vi "LED_control.vi"() -> ()   [LabVIEW 2018]
uses:
  <instrlib>/niDMM/nidmm.llb/niDMM Function.ctl
  <instrlib>/niDMM/nidmm.llb/niDMM Resolution in Digits.ctl
  <instrlib>/niDCPower/nidcpower.llb/niDCPower Measurement Type.ctl
  <vilib>/Instr/_visa.llb/VISA Configure Serial Port (Instr).vi
  <instrlib>/niDMM/nidmm.llb/niDMM Configure Measurement Digits.vi
panel:
  in  "Command":string="led_on"
  in  "Записать":bool
  in  "Tab Control":enum32{"Рабочая область", "Служебная область"}(tab)
  out "Тип индикатора":string
  in  "Питание":bool
  in  "Стоп":bool
  in  "Resource Name":refnum<k15>="PXI1Slot2" caption="Источник питания"
  in  "Мультиметр":refnum<k15>="PXI1Slot5" caption="NI DMM 1"
  in  "V_MB, V":dbl=6.0 caption="voltage level" format="%_6p"
  in  "curlim_V_MB, A":dbl=0.3 caption="current limit" format="%_6p"
  in  "curlim_V_RESERVE, A":dbl=0.1 caption="current limit" format="%_6p"
  out "currentmes_V_MB, A":dbl caption="measurement" format="%_6g"
  out "currentmes_V_RESERVE, A":dbl caption="measurement" format="%_6g"
  in  "V_RESERVE, V":dbl caption="voltage level" format="%_6p"
  out "chart_2":dbl(graph)=8.556104343922883e-07
  out "chart_0":dbl(graph)=5.42616690347781e-05 caption="Waveform Chart 5"
  in  "curlim_V_LED, A":dbl=0.03 caption="current limit" format="%_6p"
  in  "V_LED, V":dbl=2.000000000000001 caption="voltage level" format="%_6p"
  out "chart_1":dbl(graph)=2.456762028615791e-06 caption="Waveform Chart 5"
  out "currentmes_V_LED, A":dbl caption="measurement" format="%_6g"
  in  "NI DMM 1 Current Range 3":string(combo)="0,1" caption="Range"
  out "Real Current, А":dbl=1.3612861948786303e-08 format="%.5f"
  in  "NI DMM 1 units 3":string(combo)="1000" caption="Units"
  out "NI DMM 1 Current Char 3":dbl(graph)=0.013612861948786303
  out "NI DMM 1 Current 3":dbl caption="Current" format="%_6g"
  in  "Arduino":refnum<visa-resource-name>="COM14"
  in  "Сегменты":bool[](array[boolean])=[FALSE, FALSE, FALSE, FALSE, FALSE, FALSE, FALSE, FALSE, FALSE, FALSE]
  out "Разряд":dbl
  out "+/-":bool
  # "all_off - 0\nall_on - 1"
  # "j"
  # "c"
  # "d"
  # "e"
  # "g"
  # "h"
  # "a"
  # "b"
  # "f"
  # "k"
  # "L"
  # "m"
  # "n"
  # "p"
  # "dp"
  # "необходимо выдерживать 1 с между нажатиями кнопок"
  # "регулировать ток в зависимости от температуры.\nс ростом температуры растет ток.\nпид-регулятор??"
  # "\"опрашивать кнопки не чаще, чем раз в секунду. сейчас кликать можно чаще, они загорятся, но ничего не произойдет\""
  # "автоматизировать подбор напряжения по известному максимальному напряжению и току. ОС по току сегмента"
  # "регклировка суммарного тока через инлдикатор"
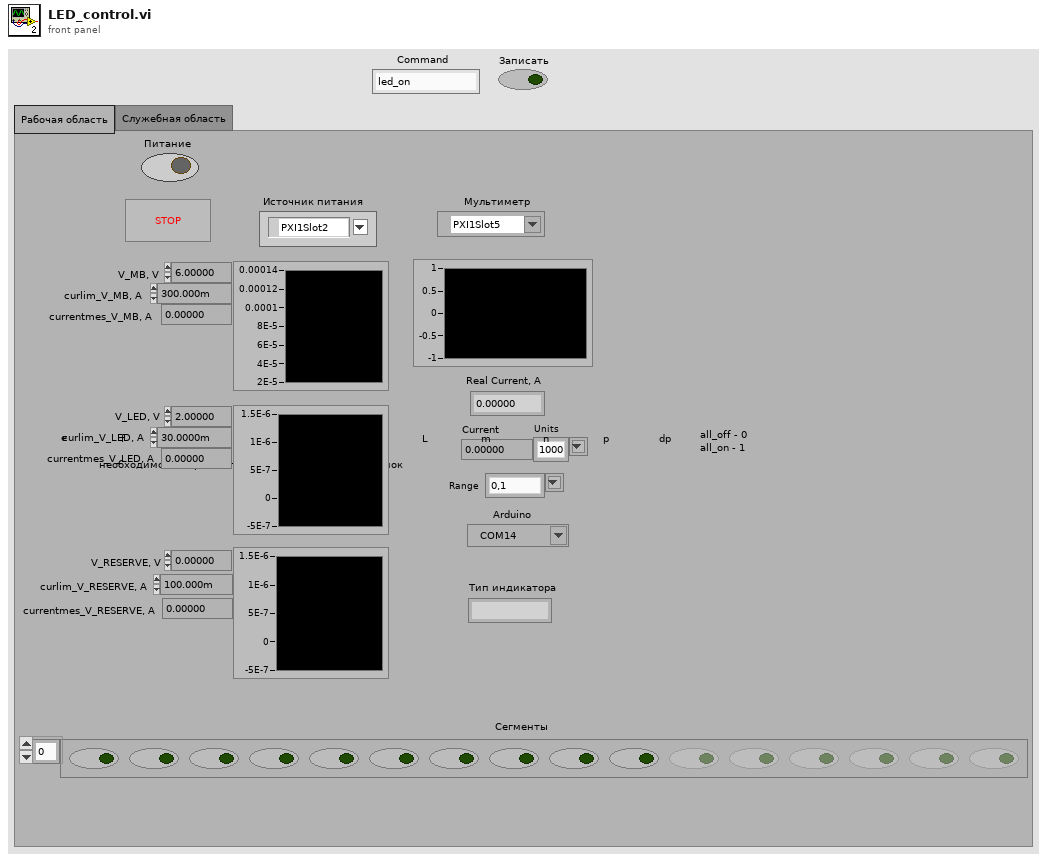
[diagram p1: front panel]
types:
  T1 = typedef "niDMM Function.ctl" = enum16{"DC Volts", "AC Volts", "DC Current", "AC Current", "2-wire Resistance", "4-wire Resistance", "Diode", "Frequency", "Period", "AC Volts DC Coupled", "Capacitance", "Inductance", "Temperature"}
  T2 = typedef "niDMM Resolution in Digits.ctl" = dbl
  T3 = typedef "niDCPower Measurement Type.ctl" = i32
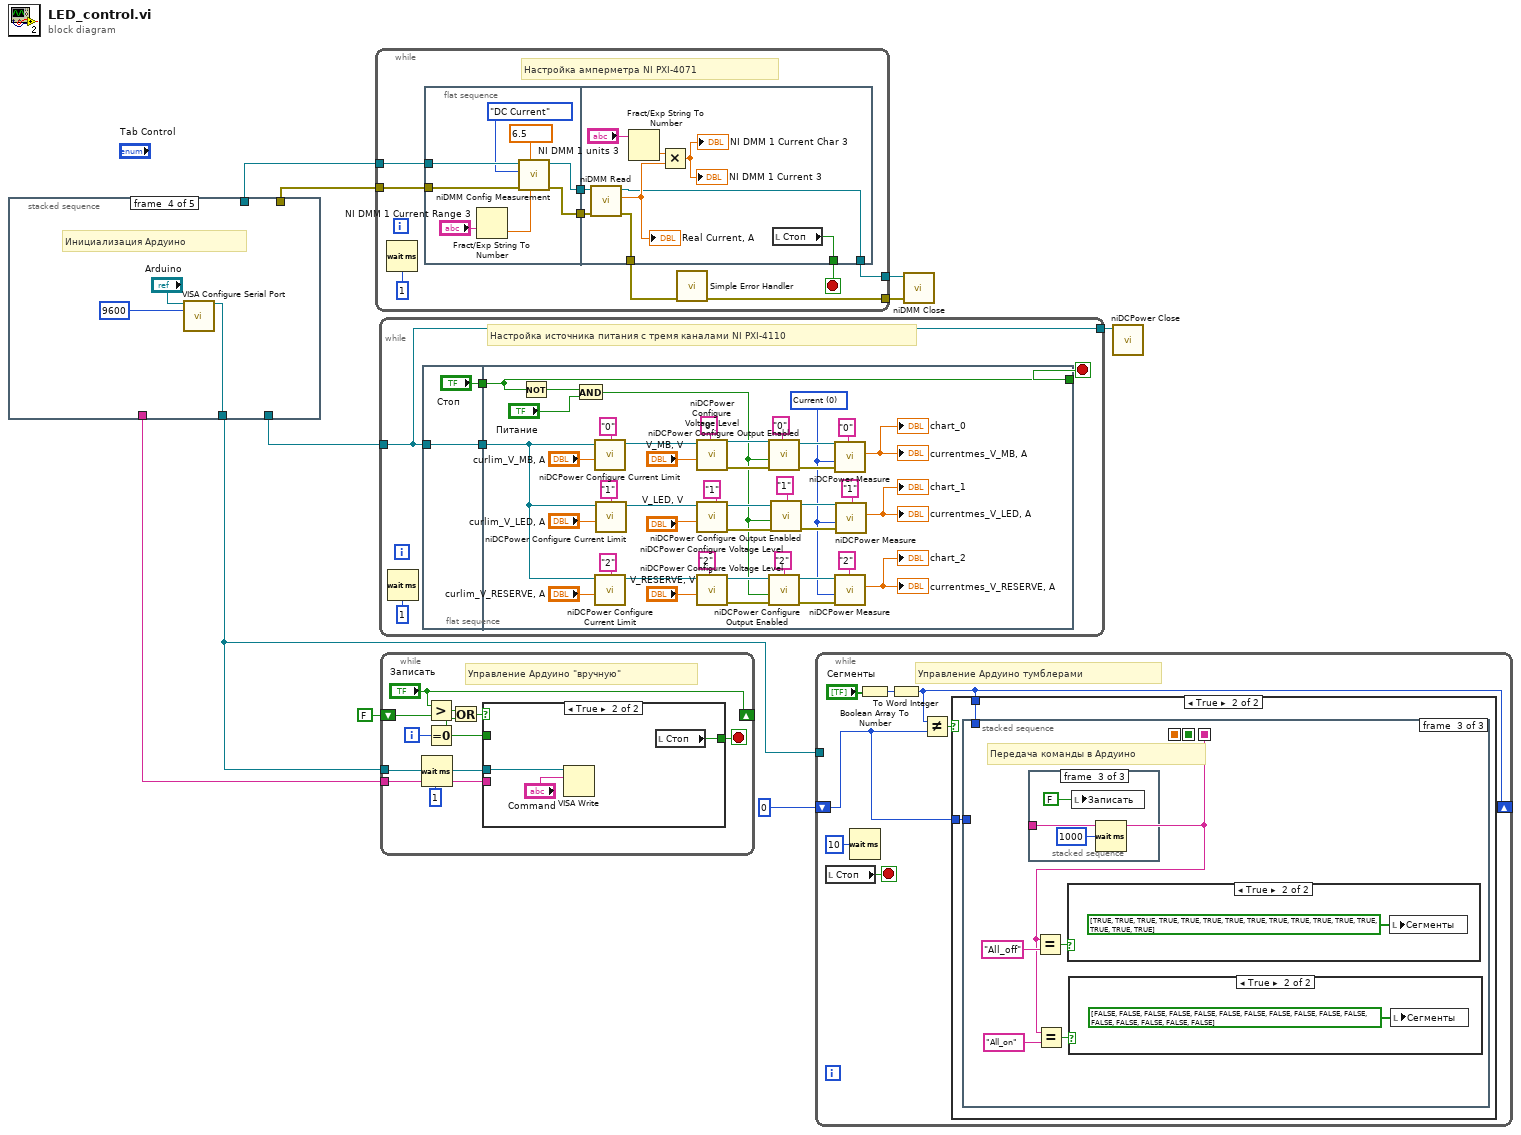
[diagram p0: block diagram]
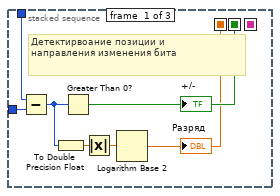
[diagram p3: hidden frame]
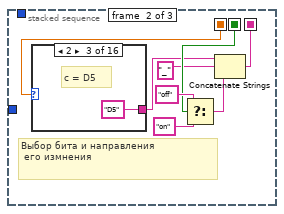
[diagram p4: hidden frame]
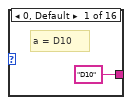
[diagram p5: hidden frame]
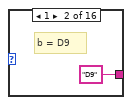
[diagram p6: hidden frame]
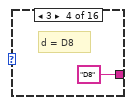
[diagram p7: hidden frame]
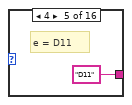
[diagram p8: hidden frame]
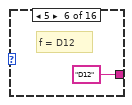
[diagram p9: hidden frame]
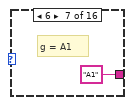
[diagram p10: hidden frame]
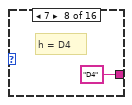
[diagram p11: hidden frame]
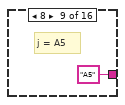
[diagram p12: hidden frame]
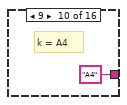
[diagram p13: hidden frame]
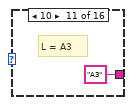
[diagram p14: hidden frame]
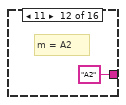
[diagram p15: hidden frame]
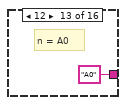
[diagram p16: hidden frame]
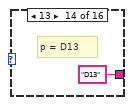
[diagram p17: hidden frame]
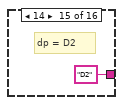
[diagram p18: hidden frame]
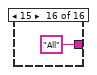
[diagram p19: hidden frame]
diagram:
  n1 = stacked-sequence {
    tunnel: [_ _ w20 _ _] -> w7
    tunnel: [_ w16 _ _ _] -> w10
    tunnel: [_ w15 _ _ _] -> w9
    tunnel: [_ _ _ w24 _] -> w4
    tunnel: [_ _ _ _ w27] -> w1
    frame #0 {
      w13 = 0.0 ("currentmes_2")
      w11 = FALSE ("Стоп")
      # "Обнуление переменных"
      n2 = local write "Питание"(w11) -> ()
      n3 = local write "Стоп"(w11) -> ()
      n4 = local write "+/-"(w11) -> ()
      n5 = local write "Сегменты"(bool[] [FALSE, FALSE, FALSE, FALSE, FALSE, FALSE, FALSE, FALSE, FALSE, FALSE] ("Сегменты")) -> ()
      n6 = local write "currentmes_V_MB, A"(w13) -> ()
      n7 = local write "currentmes_V_LED, A"(w13) -> ()
      n8 = local write "currentmes_V_RESERVE, A"(w13) -> ()
      n9 = local write "NI DMM 1 Current 3"(w13) -> ()
      n10 = local write "Разряд"(w13) -> ()
      n11 = local write "Command"("zero" ("Command 2")) -> ()
    }
    frame #1 {
      # "Инициализация амперметра"
      n12 = call <instrlib>:"niDMM Initialize.vi"("Instrument Descriptor"="Мультиметр") -> ("error out"=w16:errorcluster, "instrument handle out"=w15:refnum<k15>)  [unwired: 9 in]
    }
    frame #2 {
      # "Инициализация источника питания"
      n13 = call <instrlib>:"niDCPower Initialize.vi"("resource name"="Resource Name") -> ("error out"=w19:errorcluster, "instrument handle out"=w21:refnum<k15>)  [unwired: 3 in, 6 out]
      n14 = call <instrlib>:"niDCPower Configure Voltage Level.vi"("error in (no error)"=w19, "voltage level"=0.0, "channel name"="0,1,2", "instrument handle"=w21) -> ("instrument handle out"=w20:refnum<k15>)  [unwired: 6 in, 1 out]
    }
    frame #3 {
      # "Инициализация Ардуино"
      n15 = call-poly "VISA Configure Serial Port"("VISA resource name"="Arduino", "baud rate (9600)"=u32 9600) -> ("VISA resource name out"=w24:refnum<visa-resource-name>)  [unwired: 12 in, 1 out]
    }
    frame #4 {
      # "Всплывающее окно\nкакой индикатор?\nОА/ОК"
      n16 = call "Begin.vi"() -> ("String"=w27:string)  [unwired: 8 in]
      "Тип индикатора" <- w27
      n17 = local write "Command"(w27) -> ()
    }
  }
  n18 = while {
    tunnel: [w34] -> w2
    tunnel: w9 -> [w32]
    tunnel: w10 -> [w31]
    tunnel: [w28] -> w3
    stop <- w30 stop-if-true
    # "Настройка амперметра NI PXI-4071"
    n19 = Wait (ms)(milliseconds to wait=u32 1) -> ()  [unwired: 1 out]
    n20 = flat-sequence {
      tunnel: [w41] -> w36
      tunnel: w32 -> [w39]
      tunnel: w31 -> [w43]
      tunnel: [w40] -> w35
      tunnel: w36 -> [w49]
      tunnel: w35 -> [w52]
      tunnel: [w47] -> w30
      tunnel: [w46] -> w28
      tunnel: [w45] -> w29
      frame #0 {
        w37 = T2 6.5 items=["3 1/2"=3.5, "4 1/2"=4.5, "5 1/2"=5.5, "6 1/2"=6.5, "7 1/2"=7.5] ("Resolution in Digits")
        n21 = Fract/Exp String To Number(string="NI DMM 1 Current Range 3") -> (number=w42:dbl)  [unwired: 3 in, 1 out]
        n22 = call-poly <instrlib>:"niDMM Config Measurement.vi"("Range"=w42, "Resolution in Digits"=w37, "error in (no error)"=w43, "Function"=niDMM_Function."DC Current" ("Measurement Type"), "instrument handle"=w39) -> ("error out"=w40:errorcluster, "instrument handle out"=w41:refnum<k15>)  [unwired: 5 in]
      }
      frame #1 {
        n23 = call <instrlib>:"niDMM Read.vi"("error in (no error)"=w52, "instrument handle"=w49) -> ("error out"=w45:errorcluster, "Measurement"=w48:dbl, "instrument handle out"=w46:refnum<k15>)  [unwired: 7 in]
        "Real Current, А" <- w48
        n24 = Fract/Exp String To Number(string="NI DMM 1 units 3") -> (number=w50:dbl)  [unwired: 3 in, 1 out]
        n25 = Multiply(x=w50, y=w48) -> (x*y=→"NI DMM 1 Current 3" →"NI DMM 1 Current Char 3":dbl)
        n26 = local read "Стоп"() -> (w47:bool)
      }
    }
    n27 = call <vilib>:"Simple Error Handler.vi"("error in (no error)"=w29) -> ("error out"=w34:errorcluster)  [unwired: 1 in, 7 out]
  }
  n28 = while {
    tunnel: w7 -> [w54]
    tunnel: [w54] -> w6
    stop <- w55 stop-if-true
    # "Настройка источника питания с тремя каналами NI PXI-4110"
    n29 = Wait (ms)(milliseconds to wait=u32 1) -> ()  [unwired: 1 out]
    n30 = flat-sequence {
      tunnel: w54 -> [w60]
      tunnel: [w60] -> w57
      tunnel: ["Стоп"] -> w56
      tunnel: w57 -> [w68]
      tunnel: w56 -> [w102]
      tunnel: [w102] -> w55
      frame #0 {
      }
      frame #1 {
        w67 = T3 0 items=["Current", "Voltage"] ("measurement type")
        n31 = Not(x=w102) -> (.not. x?=w101:bool)
        n32 = And(x=w101, y="Питание") -> (x .and. y?=w63:bool)
        n33 = call <instrlib>:"niDCPower Configure Current Limit.vi"("current limit"="curlim_V_MB, A", "channel name"="0", "instrument handle"=w68) -> ("instrument handle out"=w87:refnum<k15>)  [unwired: 7 in, 1 out]
        n34 = call <instrlib>:"niDCPower Configure Current Limit.vi"("current limit"="curlim_V_RESERVE, A", "channel name"="2", "instrument handle"=w68) -> ("instrument handle out"=w86:refnum<k15>)  [unwired: 7 in, 1 out]
        n35 = call <instrlib>:"niDCPower Configure Current Limit.vi"("current limit"="curlim_V_LED, A", "channel name"="1", "instrument handle"=w68) -> ("instrument handle out"=w95:refnum<k15>)  [unwired: 7 in, 1 out]
        n36 = call <instrlib>:"niDCPower Configure Voltage Level.vi"("voltage level"="V_MB, V", "channel name"="0", "instrument handle"=w87) -> ("error out"=w92:errorcluster, "instrument handle out"=w89:refnum<k15>)  [unwired: 7 in]
        n37 = call <instrlib>:"niDCPower Configure Voltage Level.vi"("voltage level"="V_LED, V", "channel name"="1", "instrument handle"=w95) -> ("error out"=w98:errorcluster, "instrument handle out"=w96:refnum<k15>)  [unwired: 7 in]
        n38 = call <instrlib>:"niDCPower Configure Voltage Level.vi"("voltage level"="V_RESERVE, V", "channel name"="2", "instrument handle"=w86) -> ("error out"=w91:errorcluster, "instrument handle out"=w90:refnum<k15>)  [unwired: 7 in]
        n39 = call <instrlib>:"niDCPower Configure Output Enabled.vi"("error in (no error)"=w92, "output enabled"=w63, "channel name"="0", "instrument handle"=w89) -> ("error out"=w82:errorcluster, "instrument handle out"=w83:refnum<k15>)  [unwired: 6 in]
        n40 = call <instrlib>:"niDCPower Configure Output Enabled.vi"("error in (no error)"=w91, "output enabled"=w63, "channel name"="2", "instrument handle"=w90) -> ("error out"=w81:errorcluster, "instrument handle out"=w80:refnum<k15>)  [unwired: 6 in]
        n41 = call <instrlib>:"niDCPower Configure Output Enabled.vi"("error in (no error)"=w98, "output enabled"=w63, "channel name"="1", "instrument handle"=w96) -> ("error out"=w99:errorcluster, "instrument handle out"=w97:refnum<k15>)  [unwired: 6 in]
        n42 = call <instrlib>:"niDCPower Measure.vi"("error in (no error)"=w82, "measurement type"=w67, "channel name"="0", "instrument handle"=w83) -> ("measurement"=→"currentmes_V_MB, A" →"chart_0":dbl)  [unwired: 5 in, 2 out]
        n43 = call <instrlib>:"niDCPower Measure.vi"("error in (no error)"=w81, "measurement type"=w67, "channel name"="2", "instrument handle"=w80) -> ("measurement"=→"currentmes_V_RESERVE, A" →"chart_2":dbl)  [unwired: 5 in, 2 out]
        n44 = call <instrlib>:"niDCPower Measure.vi"("error in (no error)"=w99, "measurement type"=w67, "channel name"="1", "instrument handle"=w97) -> ("measurement"=→"chart_1" →"currentmes_V_LED, A":dbl)  [unwired: 5 in, 2 out]
      }
    }
  }
  n45 = while {
    tunnel: w4 -> [w108]
    shift-right: ["Записать"] -> _
    shift-left: FALSE ("Записать") -> [w110]
    tunnel: w1 -> [w106]
    i -> [w107]
    stop <- w111 stop-if-true
    # "Управление Ардуино \"вручную\""
    n46 = Wait (ms)(milliseconds to wait=u32 1) -> ()  [unwired: 1 out]
    n47 = Greater?(x="Записать", y=w110) -> (0:w104:bool)
    n48 = Equal To 0?(x=w107) -> (x = 0?=w103:bool)
    n49 = Or(x=w104, y=w103) -> (x .or. y?=w105:bool)
    n50 = case shown="True" w105 {
      tunnel: w108 -> [_ w116]
      tunnel: [w113 w115] -> w111
      tunnel: w106 -> [_ _]
      tunnel: w103 -> [_ _]
      frame False {
        n51 = local read "Стоп"() -> (w113:bool)
      }
      frame True {
        n52 = VISA Write(VISA resource name=w116, write buffer="Command") -> ()  [unwired: 1 in, 3 out]
        n53 = local read "Стоп"() -> (w115:bool)
      }
    }
  }
  n54 = while {
    shift-right: [w117] -> _
    shift-left: i16 0 -> [w119]
    tunnel: w4 -> [_]
    stop <- w123 stop-if-true
    # "Управление Ардуино тумблерами"
    n55 = local read "Стоп"() -> (w123:bool)
    n56 = Wait (ms)(milliseconds to wait=u32 10 ("millisecond timer value")) -> ()  [unwired: 1 out]
    n57 = Boolean Array To Number(Boolean array="Сегменты") -> (number=w118:u32)
    n58 = To Word Integer(number=w118) -> (16bit integer=w117:i16)
    n59 = Not Equal?(x=w117, y=w119) -> (x != y?=w120:bool)
    n60 = case shown="True" w120 {
      tunnel: w117 -> [_ w124]
      tunnel: w119 -> [_ w125]
      frame False {
      }
      frame True {
        n61 = stacked-sequence {
          seq-local: [w128 _ _] -> [_ w138 _]
          seq-local: [w126 _ _] -> [_ w133 _]
          seq-local: [_ w134 _] -> [_ _ w158]
          tunnel: w124 -> [w130 _ _]
          tunnel: w125 -> [w129 _ _]
          frame #0 {
            # "Детектирвоание позиции и\nнаправления изменения бита"
            n62 = Subtract(x=w130, y=w129) -> (x-y=w131:i16)
            n63 = To Double Precision Float(number=w131) -> (double precision float=w132:dbl)
            n64 = Greater Than 0?(x=w131) -> (x > 0?=w128:bool)
            "+/-" <- w128
            n65 = Absolute Value(x=w132) -> (abs(x)=w127:dbl)
            n66 = Logarithm Base 2(1:w127) -> (0:w126:dbl)
            "Разряд" <- w126
          }
          frame #1 {
            # "Выбор бита и направления\n его измнения"
            n67 = case shown="2" w133 {
              tunnel: ["D10" "D9" "D5" "D8" "D11" "D12" "A1" "D4" "A5" "A4" "A3" "A2" "A0" "D13" "D2" "All"] -> w136
              frame 0, Default {
                # "a = D10"
              }
              frame 1 {
                # "b = D9"
              }
              frame 2 {
                # "c = D5"
              }
              frame 3 {
                # "d = D8"
              }
              frame 4 {
                # "e = D11"
              }
              frame 5 {
                # "f = D12"
              }
              frame 6 {
                # "g = A1"
              }
              frame 7 {
                # "h = D4"
              }
              frame 8 {
                # "j = A5"
              }
              frame 9 {
                # "k = A4"
              }
              frame 10 {
                # "L = A3"
              }
              frame 11 {
                # "m = A2"
              }
              frame 12 {
                # "n = A0"
              }
              frame 13 {
                # "p = D13"
              }
              frame 14 {
                # "dp = D2"
              }
              frame 15 {
              }
            }
            n68 = Select(t="off", s=w138, f="on") -> (s? t:f=w135:string)
            n69 = Concatenate Strings(w136, "_" ("string"), w135) -> (w134:string)
          }
          frame #2 {
            # "Передача команды в Ардуино"
            n70 = stacked-sequence {
              tunnel: w158 -> [w164 _ _]
              frame #0 {
                n71 = local write "Command"(w164) -> ()
              }
              frame #1 {
                n72 = local write "Записать"(TRUE ("Записать")) -> ()
                n73 = Wait (ms)(milliseconds to wait=u32 1000) -> ()  [unwired: 1 out]
              }
              frame #2 {
                n74 = local write "Записать"(FALSE ("Записать")) -> ()
                n75 = Wait (ms)(milliseconds to wait=u32 1000) -> ()  [unwired: 1 out]
              }
            }
            n76 = Equal?(x=w158, y="All_off") -> (x = y?=w161:bool)
            n77 = Equal?(x=w158, y="All_on") -> (x = y?=w159:bool)
            n78 = case shown="True" w161 {
              frame False {
              }
              frame True {
                n79 = local write "Сегменты"(bool[] [TRUE, TRUE, TRUE, TRUE, TRUE, TRUE, TRUE, TRUE, TRUE, TRUE, TRUE, TRUE, TRUE, TRUE, TRUE, TRUE] ("Сегменты")) -> ()
              }
            }
            n80 = case shown="True" w159 {
              frame False {
              }
              frame True {
                n81 = local write "Сегменты"(bool[] [FALSE, FALSE, FALSE, FALSE, FALSE, FALSE, FALSE, FALSE, FALSE, FALSE, FALSE, FALSE, FALSE, FALSE, FALSE, FALSE] ("Сегменты")) -> ()
              }
            }
          }
        }
      }
    }
  }
  n82 = call <instrlib>:"niDMM Close.vi"("error in (no error)"=w2, "instrument handle"=w3) -> ()  [unwired: 9 in, 1 out]
  n83 = call <instrlib>:"niDCPower Close.vi"("instrument handle"=w6) -> ()  [unwired: 10 in, 1 out]
